vi "String Output Item Resize.vi"(8 "error in (no error)":errorcluster, 9 "NewBnds":T2, 10 "String UI Elements":T1, 11 "Output":T3) -> (0 "error out":errorcluster)   [LabVIEW 2015, in "OutputUI.lvclass"]
uses:
  OutputUI.lvclass
  Step/STEP_OUTPUT.ctl
  Step/OUTPUT_DATA_TYPE.ctl
  OUTPUT_CHECK_TYPE.ctl
  Step/OUTPUT_VALUE_TYPE.ctl
  <vilib>/Utility/miscctls.llb/LVRectTypeDef.ctl
  Step.lvclass
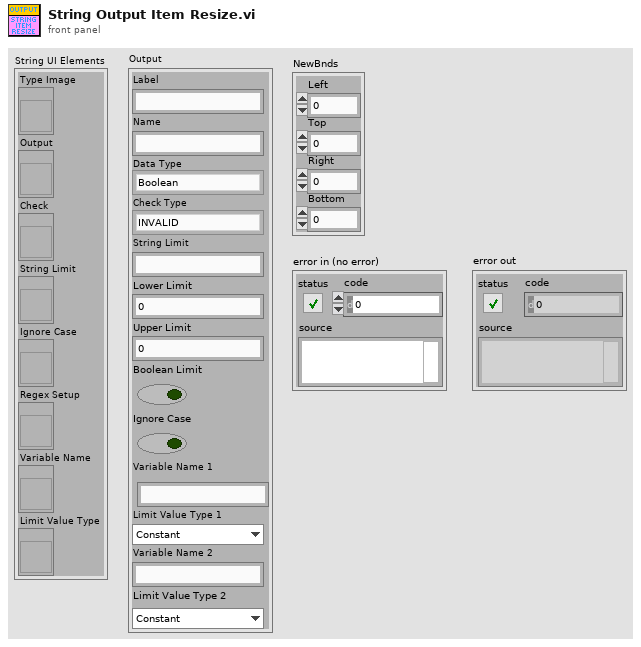
[diagram p1: front panel]
types:
  T1 = cluster{"Type Image":refnum<vi>, "Output":refnum<vi>, "Check":refnum<vi>, "String Limit":refnum<vi>, "Ignore Case":refnum<vi>, "Regex Setup":refnum<vi>, "Variable Name":refnum<vi>, "Limit Value Type":refnum<vi>}
  T2 = typedef "LVRectTypeDef.ctl" = cluster{"Left":i16, "Top":i16, "Right":i16, "Bottom":i16}
  T3 = typedef "Step.lvclass/STEP_OUTPUT.ctl" = cluster{"Label":string, "Name":string, "Data Type":T4, "Check Type":T5, "String Limit":string, "Lower Limit":dbl, "Upper Limit":dbl, "Boolean Limit":bool, "Ignore Case":bool, "Variable Name 1":string, "Limit Value Type 1":T6, "Variable Name 2":string, "Limit Value Type 2":T6}
  T4 = typedef "Step.lvclass/OUTPUT_DATA_TYPE.ctl" = enum16{"Boolean", "String", "Numeric", "Other"}
  T5 = typedef "Step.lvclass/OUTPUT_CHECK_TYPE.ctl" = enum16{"INVALID", "DO_NOT_CHECK", "RECORD", "VARIABLE", "EQUAL", "NOT_EQUAL", "STR_CONTAINS", "STR_START_WITH", "STR_END_WITH", "STR_REGEX_MATCH", "NUM_GT", "NUM_LT", "NUM_GE", "NUM_LE", "NUM_RANGE", "NUM_RANGE_BDY"}
  T6 = typedef "Step.lvclass/OUTPUT_VALUE_TYPE.ctl" = enum16{"Constant", "Variable"}
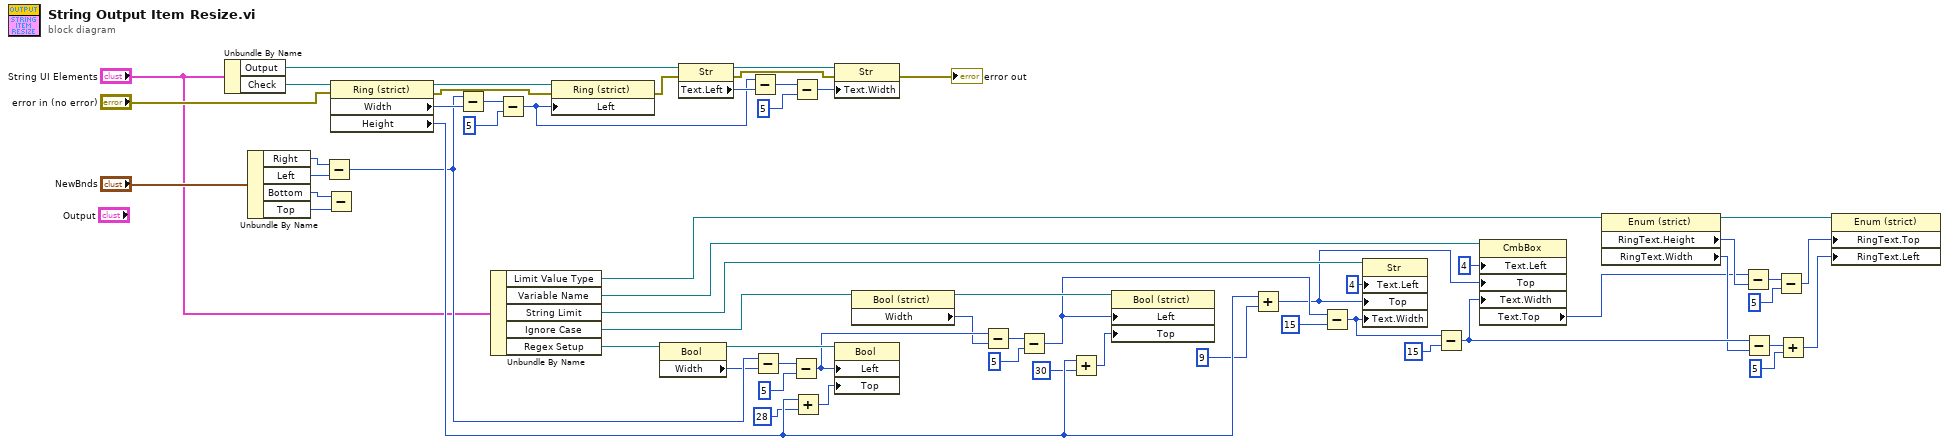
[diagram p0: block diagram]
diagram:
  n1 = Unbundle By Name("String UI Elements") -> ("Output"=w54:refnum<vi>, "Check"=w62:refnum<vi>)
  n2 = Unbundle By Name("NewBnds") -> ("Right"=w59:i16, "Left"=w60:i16, "Bottom"=w58:i16, "Top"=w57:i16)
  n3 = Subtract(x=w59, y=w60) -> (x-y=w39:i16)
  n4 = Subtract(x=w58, y=w57) -> ()  [unwired: 1 out]
  n5 = property class="Ring (strict)"(reference=w62, error in="error in (no error)") -> (reference out=w56:refnum<vi>, error out=w43:errorcluster, "Width"=w55:u32, "Height"=w40:u32)
  n6 = Subtract(x=w39, y=w55) -> (x-y=w51:u32)
  n7 = Unbundle By Name("String UI Elements") -> ("Limit Value Type"=w13:refnum<vi>, "Variable Name"=w17:refnum<vi>, "String Limit"=w22:refnum<vi>, "Ignore Case"=w30:refnum<vi>, "Regex Setup"=w37:refnum<vi>)
  n8 = Subtract(x=w51, y=5) -> (x-y=w49:u32)
  n9 = property class="Ring (strict)"(reference=w56, error in=w43, "Left"=w49) -> (error out=w42:errorcluster)  [unwired: 1 out]
  n10 = property class="Bool"(reference=w37) -> (reference out=w35:refnum<vi>, "Width"=w36:u32)  [unwired: 1 in, 1 out]
  n11 = property class="Str"(reference=w54, error in=w42) -> (reference out=w53:refnum<vi>, error out=w41:errorcluster, "Text.Left"=w52:i32)
  n12 = Subtract(x=w49, y=w52) -> (x-y=w48:u32)
  n13 = Subtract(x=w39, y=w36) -> (x-y=w34:u32)
  n14 = Subtract(x=w34, y=u32 5) -> (x-y=w29:u32)
  n15 = Subtract(x=w48, y=u32 5) -> (x-y=w47:u32)
  n16 = Add(x=w40, y=28) -> (x+y=w31:u32)
  n17 = property class="Str"(reference=w53, error in=w41, "Text.Width"=w47) -> (error out=→"error out":errorcluster)  [unwired: 1 out]
  n18 = property class="Bool"(reference=w35, "Left"=w29, "Top"=w31) -> ()  [unwired: 1 in, 2 out]
  n19 = property class="Bool (strict)"(reference=w30) -> (reference out=w25:refnum<vi>, "Width"=w28:u32)  [unwired: 1 in, 1 out]
  n20 = Subtract(x=w29, y=w28) -> (x-y=w27:u32)
  n21 = Subtract(x=w27, y=5) -> (x-y=w19:u32)
  n22 = Add(x=w40, y=30) -> (x+y=w24:u32)
  n23 = property class="Bool (strict)"(reference=w25, "Left"=w19, "Top"=w24) -> ()  [unwired: 1 in, 2 out]
  n24 = Add(x=w40, y=9) -> (x+y=w11:u32)
  n25 = Subtract(x=w19, y=u32 15) -> (x-y=w15:u32)
  n26 = property class="Str"(reference=w22, "Text.Left"=4 ("Text.Position:Left"), "Top"=w11, "Text.Width"=w15) -> ()  [unwired: 1 in, 2 out]
  n27 = Subtract(x=w15, y=u32 15) -> (x-y=w9:u32)
  n28 = property class="CmbBox"(reference=w17, "Text.Left"=4 ("Text.Position:Left"), "Top"=w11, "Text.Width"=w9) -> ("Text.Top"=w7:i32)  [unwired: 1 in, 2 out]
  n29 = property class="Enum (strict)"(reference=w13) -> (reference out=w12:refnum<vi>, "RingText.Height"=w10:u32, "RingText.Width"=w8:u32)  [unwired: 1 in, 1 out]
  n30 = Subtract(x=w7, y=w10) -> (x-y=w6:u32)
  n31 = Subtract(x=w9, y=w8) -> (x-y=w3:u32)
  n32 = Subtract(x=w6, y=u32 5) -> (x-y=w5:u32)
  n33 = Add(x=w3, y=u32 5) -> (x+y=w1:u32)
  n34 = property class="Enum (strict)"(reference=w12, "RingText.Top"=w5, "RingText.Left"=w1) -> ()  [unwired: 1 in, 2 out]
